vi "打开串口.vi"(3 "错误输入（无错误）":errorcluster, 4 "是否对话框提示？":bool, 5 "串口设置":T1={"COM号"="COM1", "波特率"=9600, "数据比特"=8, "奇偶"=enum."None", "停止位"=10, "流控制"=0} {"流控制" items=["无"=0, "XON/XOFF"=1, "RTS/CTS"=2, "DTR/DSR"=4]; "停止位" items=["1.0"=10, "1.5"=15, "2.0"=20]; "波特率" items=["75"=75, "110"=110, "134"=134, "150"=150, "300"=300, "600"=600, "1200"=1200, "1800"=1800, "2400"=2400, "4800"=4800, "7200"=7200, "9600"=9600, "14400"=14400, "19200"=19200, "28800"=28800, "38400"=38400, "56000"=56000, "57600"=57600, "115200"=115200, "128000"=128000, "230400"=230400]}) -> (0 "错误输出":errorcluster, 1 "OpenOK?":bool, 2 "串口设置输出":T1={"COM号"="", "波特率"=9600, "数据比特"=8, "奇偶"=enum."None", "停止位"=10, "流控制"=0} {"流控制" items=["无"=0, "XON/XOFF"=1, "RTS/CTS"=2, "DTR/DSR"=4]; "停止位" items=["1.0"=10, "1.5"=15, "2.0"=20]; "波特率" items=["75"=75, "110"=110, "134"=134, "150"=150, "300"=300, "600"=600, "1200"=1200, "1800"=1800, "2400"=2400, "4800"=4800, "7200"=7200, "9600"=9600, "14400"=14400, "19200"=19200, "28800"=28800, "38400"=38400, "56000"=56000, "57600"=57600, "115200"=115200, "128000"=128000, "230400"=230400]})   [LabVIEW 2015]
uses:
  Serial - Settings.ctl
  <vilib>/Instr/_visa.llb/VISA Configure Serial Port (Instr).vi
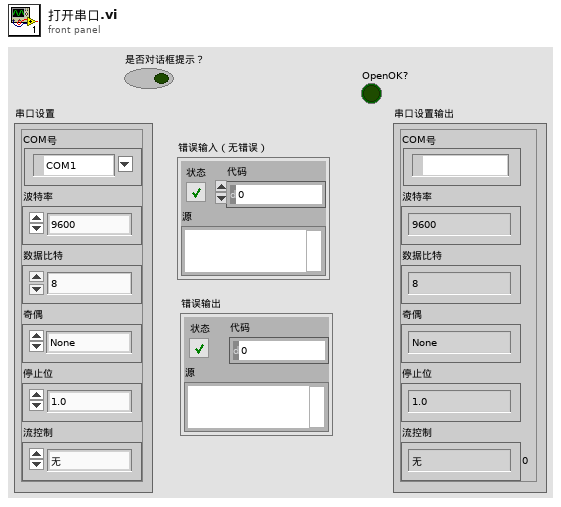
[diagram p1: front panel]
types:
  T1 = typedef "Serial - Settings.ctl" = cluster{"COM号":refnum<visa-resource-name>, "波特率":u32, "数据比特":u16, "奇偶":enum16{"None", "Odd", "Even", "Mark", "Space"}, "停止位":u16, "流控制":u16}
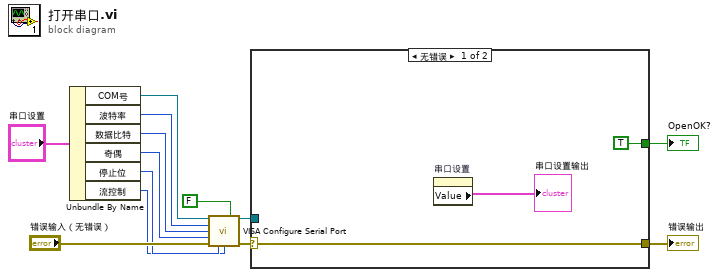
[diagram p0: block diagram]
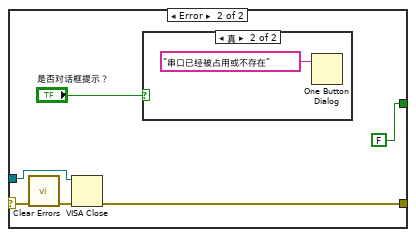
[diagram p2: hidden frame]
diagram:
  n1 = Unbundle By Name("串口设置") -> ("COM号"=w1:refnum<visa-resource-name>, "波特率"=w7:u32, "数据比特"=w8:u16, "奇偶"=w9:enum16{"None", "Odd", "Even", "Mark", "Space"}, "停止位"=w10:u16, "流控制"=w3:u16)
  n2 = call-poly "VISA Configure Serial Port"("VISA resource name"=w1, "Enable Termination\nChar (T)"=FALSE ("Enable Termination\nChar (T)"), "baud rate (9600)"=w7, "data bits (8)"=w8, "parity (0:none)"=w9, "error in (no error)"="错误输入（无错误）", "stop bits (10: 1 bit)"=w10, "flow control (0:none)"=w3) -> ("VISA resource name out"=w4:refnum<visa-resource-name>, "error out"=w6:errorcluster)  [unwired: 6 in]
  n3 = case shown="无错误" w6 {
    selector: w6 -> [w16 w22]
    tunnel: [w16 w19] -> w13
    tunnel: [TRUE ("Enable Termination\nChar (T)") FALSE ("Enable Termination\nChar (T)")] -> w5
    tunnel: w4 -> [_ w18]
    frame No Error {
      n4 = property on="串口设置" class="Clust (严格)"() -> ("Value"=→"串口设置输出":T1)  [unwired: 2 in, 2 out]
    }
    frame Error {
      n5 = call <vilib>:"Clear Errors.vi"("error in (no error)"=w22) -> ("error out"=w20:errorcluster)  [unwired: 5 in, 1 out]
      n6 = VISA Close(VISA resource name=w18, error in (no error)=w20) -> (error out=w19:errorcluster)
      n7 = case shown="真" "是否对话框提示？" {
        frame False {
        }
        frame True {
          n8 = One Button Dialog(message="串口已经被占用或不存在" ("消息")) -> ()  [unwired: 1 in, 1 out]
        }
      }
    }
  }
  "错误输出" <- w13
  "OpenOK?" <- w5
